vi "Reset Hardware List and Run Button.vi"(8 "error in (no error)":errorcluster, 11 "Measurement UI in":refnum<class "Measurement UI.lvclass">) -> (0 "error out":errorcluster, 3 "Measurement UI out":refnum<class "Measurement UI.lvclass">)   [LabVIEW 2016, in "Measurement UI.lvlib" / "Measurement UI.lvclass"]
uses:
  Measurement UI.lvclass
  Measurement UI.lvclass/Measurement UI.ctl
  Read Run Indefinitely.vi
  Accessors/Read Show FP_.vi
  Accessors/Read Run.vi
  Accessors/Read Step Iterations.vi
  Accessors/Read Digitizer.vi
  Read Multimeter.vi
  Accessors/Read Function Generator.vi
  Accessors/Read Power Supply.vi
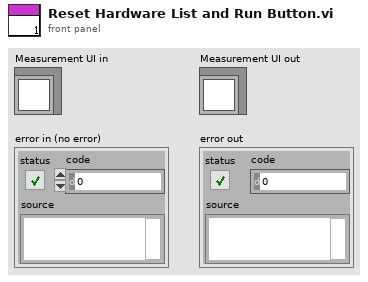
[diagram p1: front panel]
types:
  T1 = enum8{"Enabled", "Disabled", "Disabled and Grayed Out"}
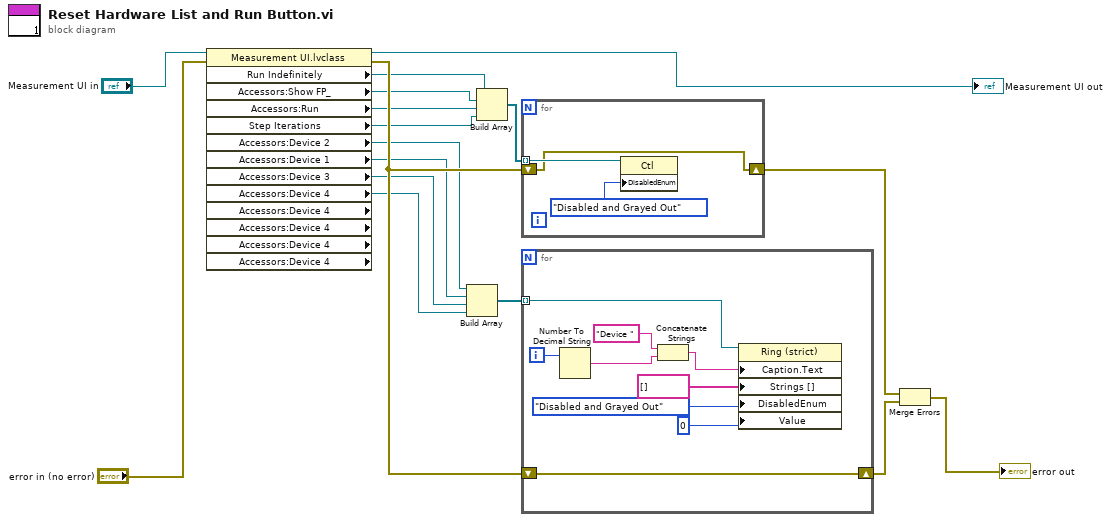
[diagram p0: block diagram]
diagram:
  n1 = property class="Measurement UI.lvclass" props=["Run Indefinitely", "Accessors:Show FP_", "Accessors:Run", "Step Iterations", "Accessors:Device 2", "Accessors:Device 1", "Accessors:Device 3", "Accessors:Device 4", "Accessors:Device 4", "Accessors:Device 4", "Accessors:Device 4", "Accessors:Device 4"](reference="Measurement UI in", error in="error in (no error)") -> (reference out=→"Measurement UI out":refnum<class "Measurement UI.lvclass">, error out=w14:errorcluster, "Run Indefinitely"=w1:refnum<vi>, "Accessors:Show FP_"=w2:refnum<vi>, "Accessors:Run"=w4:refnum<vi>, "Step Iterations"=w5:refnum<vi>, "Accessors:Device 2"=w8:refnum<vi>, "Accessors:Device 1"=w9:refnum<vi>, "Accessors:Device 3"=w10:refnum<vi>, "Accessors:Device 4"=w11:refnum<vi>)  [unwired: 4 out]
  n2 = Build Array(w8, w9, w10, w11) -> (w6:refnum<vi>[])
  n3 = Build Array(w1, w2, w4, w5) -> (w3:refnum<vi>[])
  n4 = for {
    tunnel: w3 -> [w20] mode=indexing
    shift-right: [w18] -> w16
    shift-left: w14 -> [w18]
    n5 = property class="Ctl"(reference=w20, "DisabledEnum"=T1."Disabled and Grayed Out" ("Disabled")) -> ()  [unwired: 1 in, 2 out]
  }
  n6 = for {
    tunnel: w6 -> [w26] mode=indexing
    shift-right: [w21] -> w15
    shift-left: w14 -> [w21]
    i -> [w25]
    n7 = Number To Decimal String(number=w25) -> (decimal integer string=w23:string)  [unwired: 1 in]
    n8 = Concatenate Strings("Device ", w23) -> (w22:string)
    n9 = property class="Ring (strict)"(reference=w26, "Caption.Text"=w22, "Strings []"=string[] [], "DisabledEnum"=T1."Disabled and Grayed Out" ("Disabled"), "Value"=u16 0) -> ()  [unwired: 1 in, 2 out]
  }
  n10 = Merge Errors(w16, w15) -> (→"error out":errorcluster)
